vi "Listen and reply broadcast.ping (subVi).vi"(2 "error (in)":errorcluster, 3 "host name":string="higgsino.physics.ucsb.edu") -> (0 "error out":errorcluster, 1 "Log":string)   [LabVIEW 2016]
uses:
  C:/Program Files (x86)/National Instruments/LabVIEW 2016/vi.lib/Distrio/LabbitMQ/RabbitMQ.Client.dll
  Program Files (x86)/National Instruments/LabVIEW 2016/vi.lib/Distrio/LabbitMQ/RabbitMQ.Client.dll
  <vilib>/Distrio/LabbitMQ/Queue/Queue.lvclass
  <vilib>/Distrio/LabbitMQ/Connection/Connection.lvclass
panel:
  in  "stop":bool
  in  "Tab Control":enum32{"AMQP Settings", "Logger"}(tab)
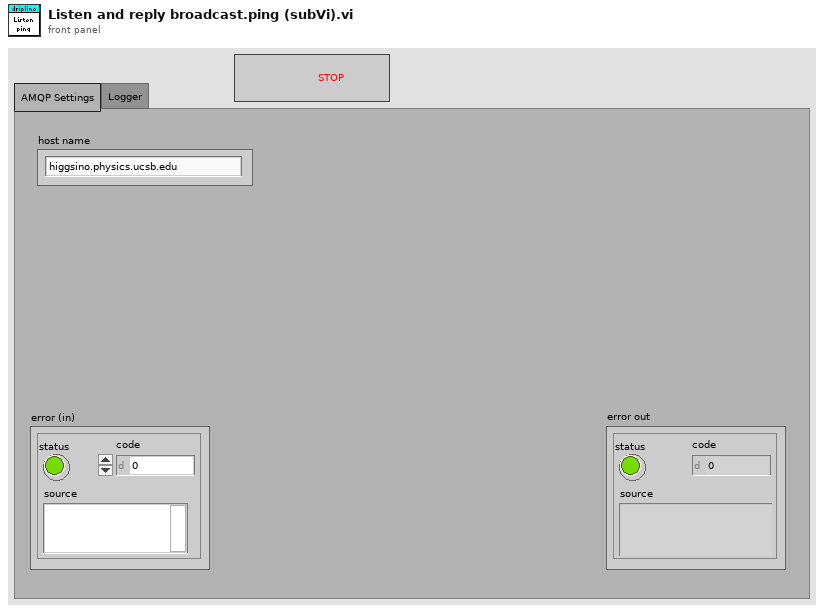
[diagram p1: front panel]
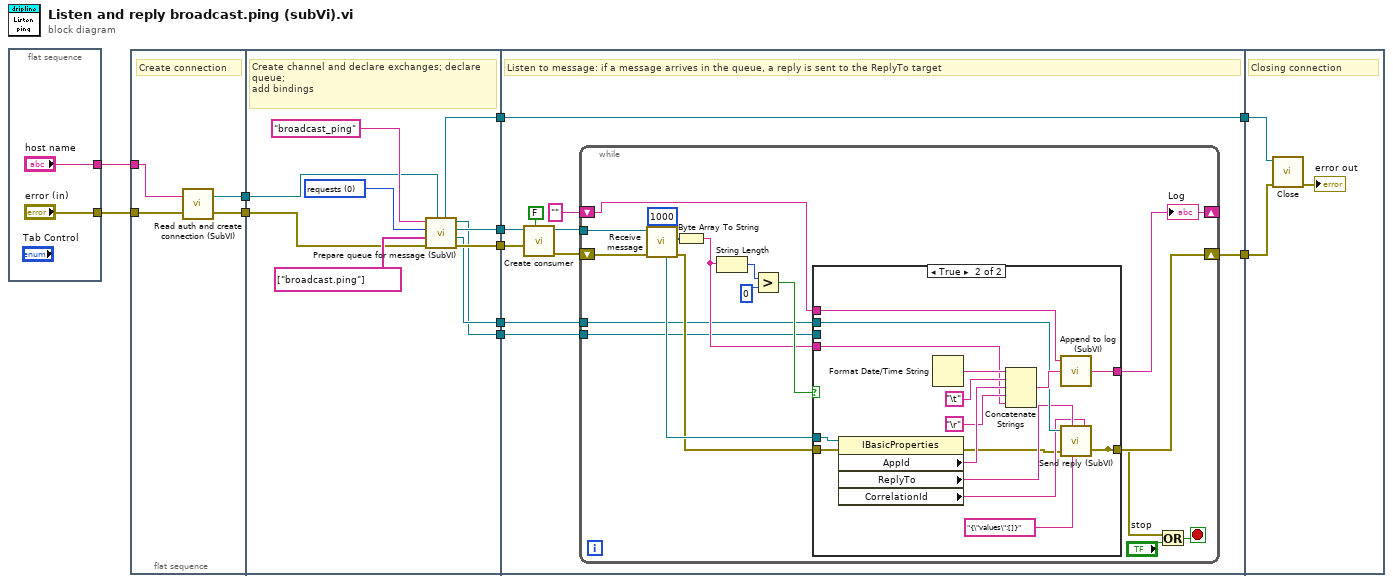
[diagram p0: block diagram]
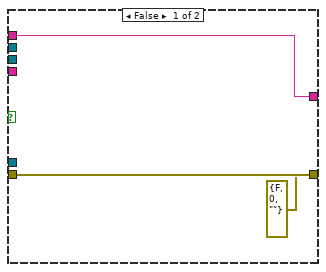
[diagram p2: hidden frame]
diagram:
  n1 = flat-sequence {
    tunnel: ["error (in)"] -> w9
    tunnel: ["host name"] -> w8
    frame #0 {
    }
  }
  n2 = flat-sequence {
    tunnel: [w15] -> w11
    tunnel: [w14] -> w10
    tunnel: w8 -> [w17]
    tunnel: w9 -> [w16]
    tunnel: w11 -> [w22]
    tunnel: w10 -> [w21]
    tunnel: [w24] -> w6
    tunnel: [w23] -> w5
    tunnel: [w20] -> w3
    tunnel: [w19] -> w2
    tunnel: [w18] -> w1
    tunnel: [w36] -> w7
    tunnel: w6 -> [w33]
    tunnel: w5 -> [w32]
    tunnel: [w31] -> w4
    tunnel: w3 -> [w31]
    tunnel: w2 -> [w30]
    tunnel: w1 -> [w29]
    tunnel: w7 -> [w76]
    tunnel: w4 -> [w75]
    frame #0 {
      # "Create connection"
      n3 = call "Read auth and create connection (SubVI).vi"("error in (no error)"=w16, "host name"=w17) -> ("error out"=w14:errorcluster, "Connection out"=w15:refnum<class "Connection.lvclass">)
    }
    frame #1 {
      w25 = u16 0 items=["requests", "alerts"] ("exchange name")
      # "Create channel and declare exchanges; declare queue;\nadd bindings"
      n4 = call "Prepare queue for message (SubVI).vi"("Connection in"=w22, "error in (no error)"=w21, "binding key"=string[] ["broadcast.ping"] ("broadcast.ping"), "exchange name"=w25, "queue \nname"="broadcast_ping" ("queue name")) -> ("error out"=w23:errorcluster, "Exchange.lvclass"=w19:refnum<class "Exchange.lvclass">, "Queue out"=w24:refnum<class "Queue.lvclass">, "Channel out"=w18:refnum<class "Channel.lvclass">, "Connection out"=w20:refnum<class "Connection.lvclass">)
    }
    frame #2 {
      # "Listen to message: if a message arrives in the queue, a reply is sent to the ReplyTo target"
      n5 = call <vilib>:"Create consumer.vi"("noAck? (T)"=FALSE, "error in (no error)"=w32, "Queue in"=w33) -> ("error out"=w35:errorcluster, "Queue out"=w37:refnum<class "Queue.lvclass">)  [unwired: 7 in]
      n6 = while {
        tunnel: w37 -> [w55]
        shift-right: [w47] -> w36
        shift-left: w35 -> [w54]
        shift-right: [w51] -> _
        shift-left: "" -> [w52]
        tunnel: w30 -> [w39]
        tunnel: w29 -> [w38]
        stop <- w40 stop-if-true
        n7 = call <vilib>:"Receive message.vi"("millisecondsTimeout"=1000, "error in (no error)"=w54, "Consumer in"=w55) -> ("error out"=w49:errorcluster, "message body"=w53:u8[], "MessageProperties"=w50:refnum<k24>)  [unwired: 3 in, 3 out]
        n8 = Byte Array To String(unsigned byte array=w53) -> (string=w41:string)
        n9 = String Length(string=w41) -> (length=w44:i32)
        n10 = Greater?(x=w44, y=0) -> (0:w42:bool)
        n11 = case shown="True" w42 {
          tunnel: w52 -> [w58 w74]
          tunnel: [w58 w73] -> w51
          tunnel: w50 -> [_ w72]
          tunnel: w41 -> [_ w67]
          tunnel: w49 -> [w57 w65]
          tunnel: [w57 w59] -> w47
          tunnel: [errorcluster {"status"=FALSE, "code"=0, "source"=""} ("error out") w59] -> w46
          tunnel: w39 -> [_ w64]
          tunnel: w38 -> [_ _]
          frame False {
          }
          frame True {
            n12 = property class="IBasicProperties"(reference=w72, error in=w65) -> (error out=w60:errorcluster, "AppId"=w69:string, "ReplyTo"=w63:string, "CorrelationId"=w62:string)  [unwired: 1 out]
            n13 = Format Date/Time String() -> (date/time string=w71:string)  [unwired: 3 in]
            n14 = Concatenate Strings(w71, "\t", w69, "\r", w67) -> (w66:string)
            n15 = call "Append to log (SubVI).vi"("to append"=w66, "log in"=w74) -> ("log out"=w73:string)  [unwired: 1 in]
            n16 = call "Send reply (SubVI).vi"("Exchange.lvclass"=w64, "target"=w63, "error in (no error)"=w60, "reply content"="{\"values\":[]}", "Correlation ID"=w62) -> ("error out"=w59:errorcluster)  [unwired: 1 in]
          }
        }
        "Log" <- w51
        n17 = Or(x=w46, y="stop") -> (x .or. y?=w40:bool)
      }
    }
    frame #3 {
      # "Closing connection"
      n18 = call <vilib>:"Close.vi"("error in (no error)"=w76, "Connection in"=w75) -> ("error out"=→"error out":errorcluster)  [unwired: 8 in, 1 out]
    }
  }
